vi "Zero Velocity.vi"() -> ()   [LabVIEW 2019]
panel:
  out "Zero Velocity?":bool
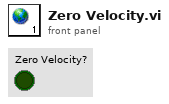
[diagram p1: front panel]
diagram:
